vi "CheckValidReference.vi"(8 "error in":errorcluster, 11 "message ref in":refnum<class "CLM_LocalMessage.lvclass">) -> (0 "error out":errorcluster, 2 "valid?":bool, 3 "message ref out":refnum<class "CLM_LocalMessage.lvclass">)   [LabVIEW 2013, in "CLM_LocalMessage.lvclass"]
uses:
  CLM_LocalMessage.lvclass
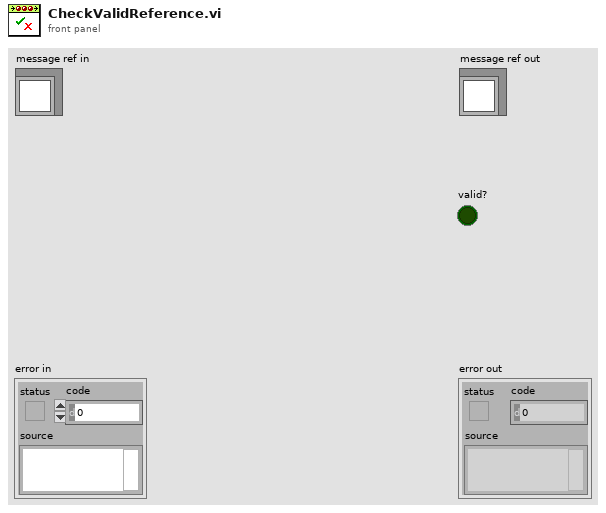
[diagram p1: front panel]
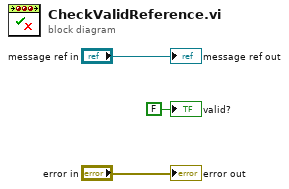
[diagram p0: block diagram]
diagram:
  "error out" <- "error in"
  "message ref out" <- "message ref in"
  "valid?" <- FALSE ("valid?")
